vi "PythonNodeForTelloVideoTester.vi"() -> ()   [LabVIEW 2018]
panel:
  in  "stop":bool
  out "iteration":i32
  out "Tello image":T1(plugin-control)
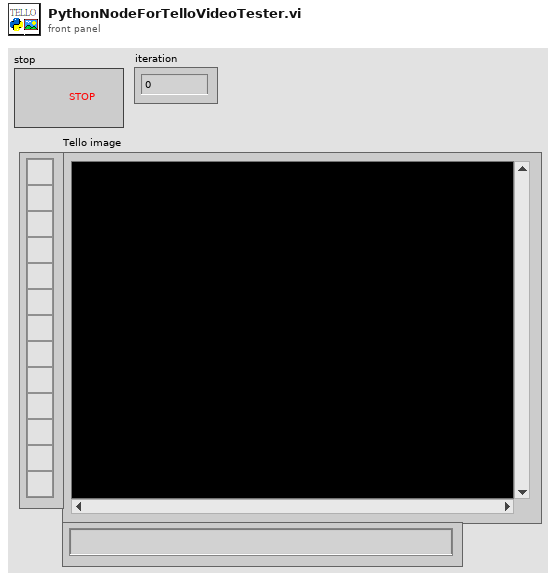
[diagram p1: front panel]
types:
  T1 = typedef "IMAQ Image.ctl" = refnum<image>
  T2 = typedef "Image Type" = u32
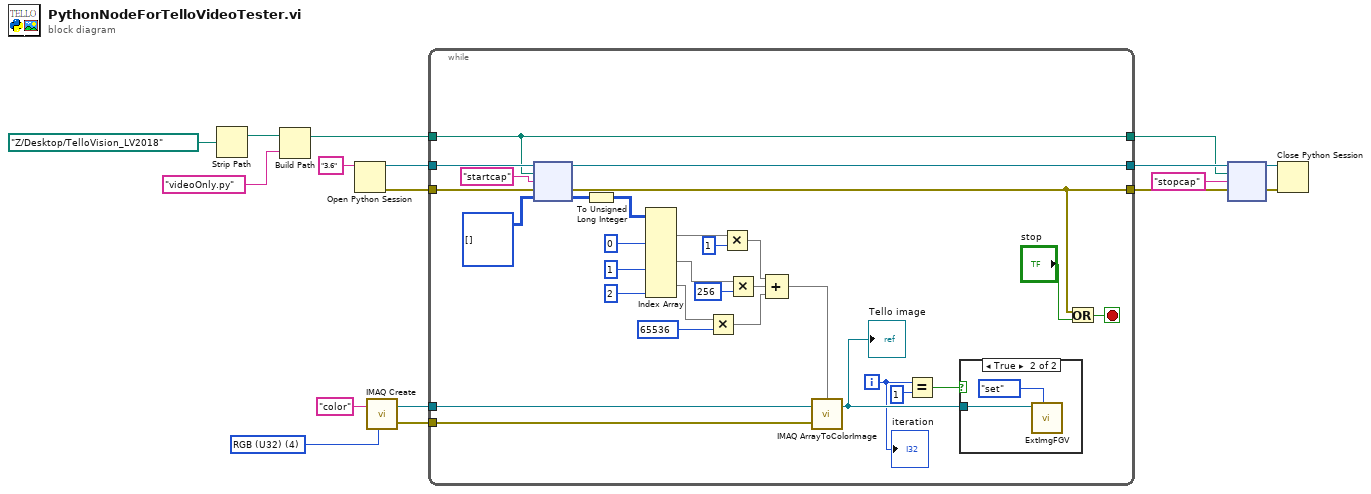
[diagram p0: block diagram]
diagram:
  w8 = T2 4 items=["Grayscale (U8)", "Grayscale (I16)", "Grayscale (SGL)", "Complex (CSG)", "RGB (U32)", "HSL (U32)", "RGB (U64)", "Grayscale (U16)"] ("Image Type")
  n1 = Strip Path(path=path "Z:/Desktop/TelloVision_LV2018") -> (stripped path=w6:path)  [unwired: 1 out]
  n2 = Build Path(base path=w6, name or relative path="videoOnly.py") -> (appended path=w4:path)
  n3 = Open Python Session(python version="3.6" ("Python version")) -> (session out=w16:refnum<k35>, error out=w15:errorcluster)  [unwired: 2 in]
  n4 = call "IMAQ Create"("Image Name"="color", "Image Type"=w8) -> ("New Image"=w7:T1, "error out"=w2:errorcluster)  [unwired: 3 in]
  n5 = while {
    tunnel: [w45] -> w14
    tunnel: [w23] -> w10
    tunnel: w16 -> [w26]
    tunnel: w15 -> [w25]
    tunnel: w7 -> [w29]
    tunnel: w4 -> [w20]
    tunnel: w2 -> [w22]
    tunnel: [w20] -> w1
    i -> [w19]
    stop <- w21 stop-if-true
    n6 = node(w26, w20, "startcap" ("function name"), w25, u8[][][] []) -> (w45:refnum<k35>, w23:errorcluster, w44:u8[][][])  [unwired: 2 out]
    n7 = To Unsigned Long Integer(number=w44) -> (unsigned 32bit integer=w30:u32[][][])
    n8 = Index Array(array=w30, index (dim 2) #1=0 ("disabled index (col)"), index (dim 2) #2=1 ("index (col)"), index (dim 2) #3=2 ("index (col)")) -> (element #1=w40:u32[][], element #2=w38:u32[][], element #3=w32:u32[][])  [unwired: 6 in]
    n9 = Multiply(x=w32, y=u32 65536) -> (x*y=w31:u32[][])
    n10 = Multiply(x=w40, y=u32 1) -> (x*y=w36:u32[][])
    n11 = Multiply(x=w38, y=u32 256) -> (x*y=w35:u32[][])
    n12 = Compound Arithmetic op=ADD(w36, w35, w31) -> (w34:u32[][])
    n13 = call "IMAQ ArrayToColorImage"("Image Pixels (U32)"=w34, "Image"=w29, "error in (no error)"=w22) -> ("Image Out"=w27:T1)  [unwired: 2 in, 1 out]
    "Tello image" <- w27
    n14 = Equal?(x=w19, y=1 ("x")) -> (x = y?=w28:bool)
    n15 = case shown="True" w28 {
      tunnel: w27 -> [_ w49]
      frame False {
      }
      frame True {
        n16 = call "ExtImgFGV.vi"("Enum"=enum16{"set", "read", "close"}."set", "Image In"=w49) -> ()  [unwired: 8 in, 2 out]
      }
    }
    n17 = Or(x=w23, y="stop") -> (x .or. y?=w21:bool)
    "iteration" <- w19
  }
  n18 = node(w14, w1, "stopcap" ("function name"), w10) -> (w11:refnum<k35>, w12:errorcluster)  [unwired: 2 in, 2 out]
  n19 = Close Python Session(session in=w11, error in=w12) -> ()  [unwired: 1 out]
